vi "Update DeviceID Array.vi"(8 "error in":errorcluster, 10 "DeviceID Array":T1[](array[typedef]), 11 "Master Controller in":refnum<class "EMS User Interface.lvclass">) -> (0 "error out":errorcluster, 3 "Master Controller out":refnum<class "EMS User Interface.lvclass">)   [LabVIEW 2018, in "EMS User Interface Actor.lvlib" / "EMS User Interface.lvclass"]
uses:
  EMS User Interface.lvclass
  <vilib>/ORNL/CSEISMIC DDS/CSEISMIC DDS Base/Data Types/Controls/DeviceID.ctl
  EMS User Interface.lvclass/EMS User Interface.ctl
  Dialog Actors/Devices to Load Actor/Devices to Load Messages/Update Device List Msg/Update Device List Msg.lvclass/Update Device List Msg.ctl
  <vilib>/ActorFramework/Message Enqueuer/Message Enqueuer.lvclass/Message Enqueuer.ctl
  Dialog Actors/VF Device Selection Actor/VF Device Selection Messages/Update Device List Msg/Update Device List Msg.lvclass/Update Device List Msg.ctl
  <vilib>/ActorFramework/Message Enqueuer/Enqueue.vi
  Dialog Actors/Devices to Load Actor/Devices to Load Messages/Update Device List Msg/Update Device List Msg.lvclass
  C:/Program Files (x86)/National Instruments/LabVIEW 2018/vi.lib/ActorFramework/Message/Message.lvclass
  Dialog Actors/VF Device Selection Actor/VF Device Selection Messages/Update Device List Msg/Update Device List Msg.lvclass
  <vilib>/ActorFramework/Message Priority Queue/Priority Enqueue.vi
  <vilib>/ORNL/CSEISMIC DDS/CSEISMIC DDS Base/CSEISMIC DDS.lvclass
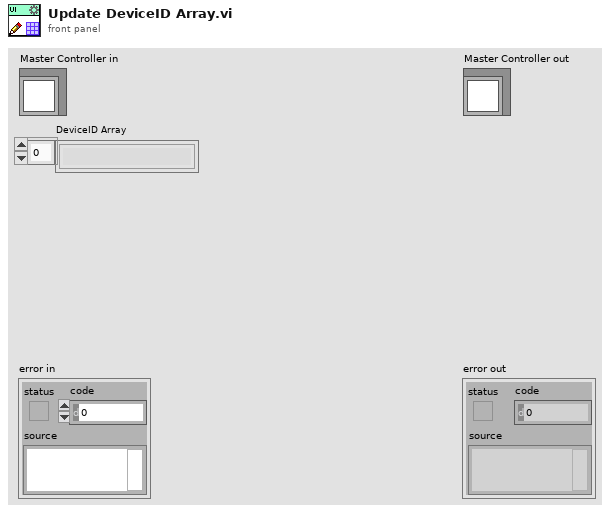
[diagram p1: front panel]
types:
  T1 = typedef "CSEISMIC DDS.lvlib/CSEISMIC DDS.lvclass/DeviceID.ctl" = string
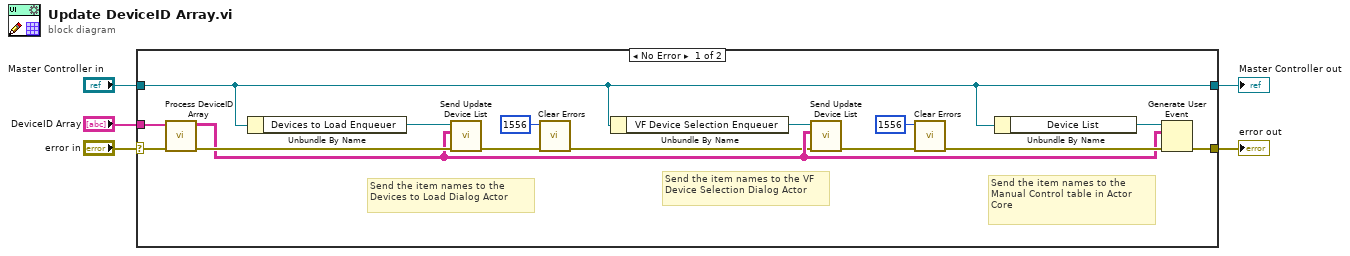
[diagram p0: block diagram]
diagram:
  n1 = case shown="No Error" "error in" {
    selector: "error in" -> [w18 w22]
    tunnel: [w15 w22] -> w4
    tunnel: [w12 w21] -> w2
    tunnel: "Master Controller in" -> [w12 w21]
    tunnel: "DeviceID Array" -> [w13 _]
    frame No Error {
      # "Send the item names to the VF Device Selection Dialog Actor"
      # "Send the item names to the Manual Control table in Actor Core"
      # "Send the item names to the Devices to Load Dialog Actor"
      n2 = call "Process DeviceID Array.vi"("error in"=w18, "DeviceID Array"=w13) -> ("error out"=w17:errorcluster, "Array"=w10:T1[][])  [unwired: 8 in]
      n3 = Unbundle By Name(w12) -> ("Devices to Load Enqueuer"=w19:refnum<class "Message Enqueuer.lvclass">)
      n4 = call "Send Update Device List.vi"("error in"=w17, "Device Table Strings"=w10, "Message Enqueuer"=w19) -> ("error out"=w7:errorcluster)  [unwired: 7 in, 1 out]
      n5 = call <vilib>:"Clear Errors.vi"("error in (no error)"=w7, "specific error code to clear (0: all)"=1556) -> ("error out"=w6:errorcluster)  [unwired: 4 in, 1 out]
      n6 = Unbundle By Name(w12) -> ("VF Device Selection Enqueuer"=w11:refnum<class "Message Enqueuer.lvclass">)
      n7 = call "Send Update Device List.vi"("error in"=w6, "Device Table Strings"=w10, "Message Enqueuer"=w11) -> ("error out"=w9:errorcluster)  [unwired: 7 in, 1 out]
      n8 = call <vilib>:"Clear Errors.vi"("error in (no error)"=w9, "specific error code to clear (0: all)"=1556) -> ("error out"=w16:errorcluster)  [unwired: 4 in, 1 out]
      n9 = Unbundle By Name(w12) -> ("Device List"=w14:refnum<user-event>)
      n10 = Generate User Event(user event=w14, event data cluster=w10, error in=w16) -> (error out=w15:errorcluster)  [unwired: 1 in, 1 out]
    }
    frame Error {
    }
  }
  "error out" <- w4
  "Master Controller out" <- w2
